vi "Get Power Waveform.vi"(9 "Config":T1={"Voltage Index"=1, "Current Index"=2, "Channel name"="Source-Current"}, 11 "array":waveform(dbl)[](array[waveform])) -> (1 "Voltage channel name":string, 3 "waveform out":waveform(dbl))   [LabVIEW 2019]
doc: "This example demonstrates how to acquire a continuous amount of data (Waveform) using the DAQ device's internal clock. It also shows how to synchronize two devices for different device families (E Series, S Series, M Series, X Series, DSA, and SC Express), to simultaneously acquire the data.\n\nFor instructions on how to connect your signals to the DAQ device, refer to your device documentation."
panel:
  out "Current channel name":string
  # "Get Power Waveform"
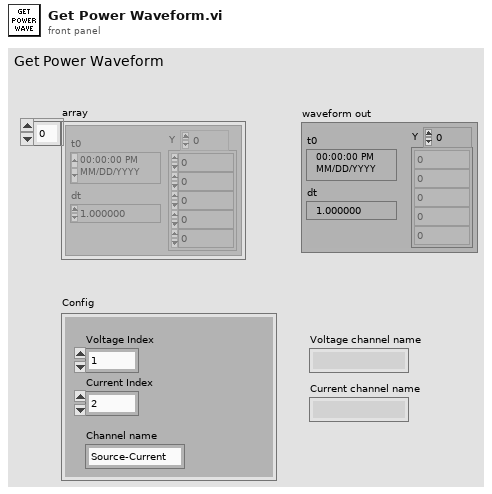
[diagram p1: front panel]
types:
  T1 = cluster{"Voltage Index":i32, "Current Index":i32, "Channel name":string}
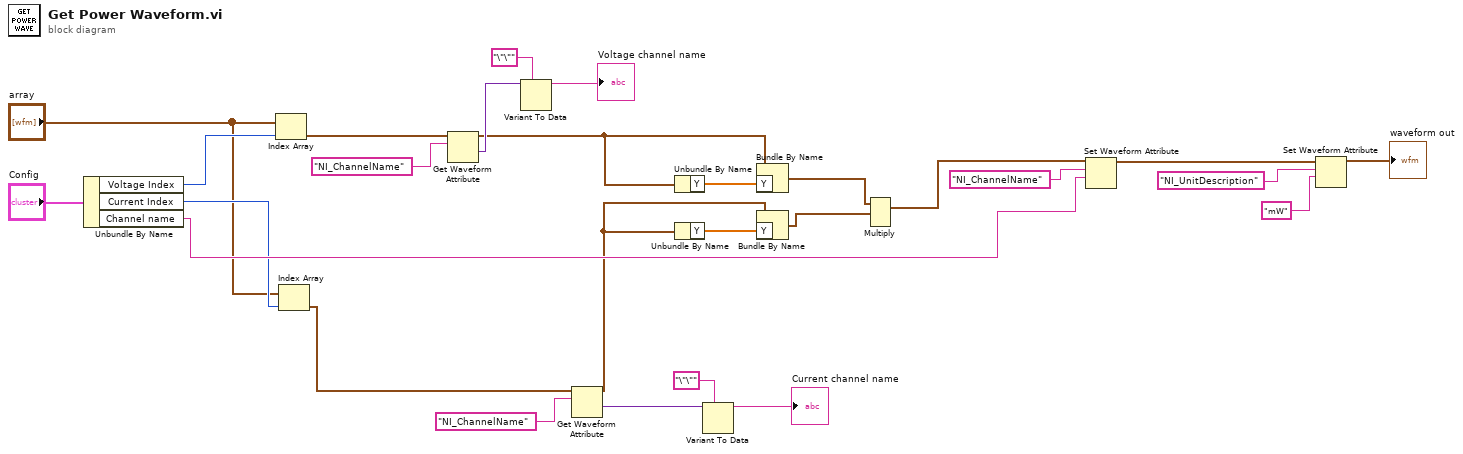
[diagram p0: block diagram]
diagram:
  n1 = Unbundle By Name("Config") -> ("Voltage Index"=w19:i32, "Current Index"=w11:i32, "Channel name"=w13:string)
  n2 = Index Array(array="array", index=w19) -> (element=w23:waveform(dbl))
  n3 = Index Array(array="array", index=w11) -> (element=w6:waveform(dbl))
  n4 = Get Waveform Attribute(6:"NI_ChannelName" ("name"), 7:w23) -> (1:w17:variant, 3:w15:waveform(dbl))  [unwired: 2 in, 2 out]
  n5 = Variant To Data(type="\"\"" ("name"), Variant=w17) -> (data=→"Voltage channel name":string)  [unwired: 1 in, 1 out]
  n6 = Get Waveform Attribute(6:"NI_ChannelName" ("name"), 7:w6) -> (1:w7:variant, 3:w1:waveform(dbl))  [unwired: 2 in, 2 out]
  n7 = Unbundle By Name(w15) -> ("Y"=w14:dbl[])
  n8 = Unbundle By Name(w1) -> ("Y"=w3:dbl[])
  n9 = Variant To Data(type="\"\"" ("name"), Variant=w7) -> (data=→"Current channel name":string)  [unwired: 1 in, 1 out]
  n10 = Bundle By Name(cluster=w15, "Y"=w14) -> (w4:waveform(dbl))
  n11 = Bundle By Name(cluster=w1, "Y"=w3) -> (w2:waveform(dbl))
  n12 = Multiply(1:w2, 2:w4) -> (0:w12:waveform(dbl))  [unwired: 1 in, 1 out]
  n13 = Set Waveform Attribute(5:w13, 6:"NI_ChannelName" ("name"), 7:w12) -> (3:w25:waveform(dbl))  [unwired: 1 in, 2 out]
  n14 = Set Waveform Attribute(5:"mW" ("name"), 6:"NI_UnitDescription" ("name"), 7:w25) -> (3:→"waveform out":waveform(dbl))  [unwired: 1 in, 2 out]
